vi "drive_to_wall.vi"(11 "NXT":T1) -> (3 "NXT 2":T1 caption="NXT")   [LabVIEW 2012]
uses:
  <vilib>/NXT/Subs/LVHSConnector.ctl
  <vilib>/NXT/Subs/MotorOutput.ctl
  <vilib>/NXT/Block Support/NXT_InputPort.ctl
  <vilib>/NXT/Dual Mode Library/Motors/MotorBrake.vi
  <vilib>/NXT/Dual Mode Library/prims/addArrayElements_int.vi
  <vilib>/NXT/Dual Mode Library/Motors/MotorReverse.vi
  <vilib>/NXT/Dual Mode Library/Waits/Wait_Num(msec).vi
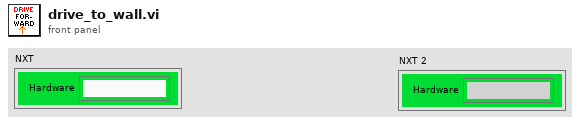
[diagram p1: front panel]
types:
  T1 = typedef "LVHSConnector.ctl" = cluster{"Hardware":string, "Flattened String":string}
  T2 = typedef "MotorOutput.ctl" = u8
  T3 = typedef "NXT_InputPort.ctl" = u8
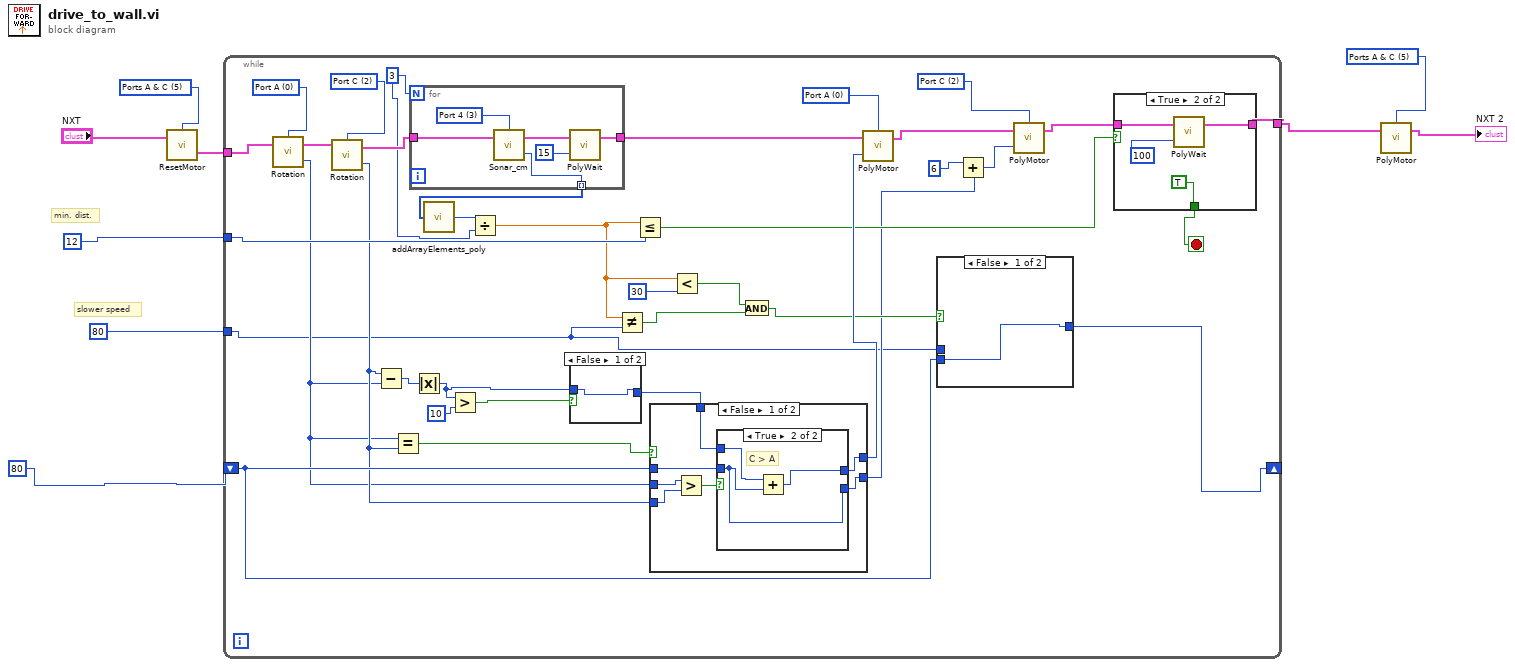
[diagram p0: block diagram]
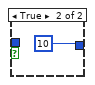
[diagram p2: hidden frame]
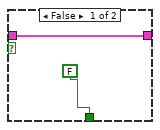
[diagram p4: hidden frame]
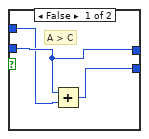
[diagram p5: hidden frame]
diagram:
  w9 = T2 5 items=["Port A"=0, "Port B"=1, "Port C"=2, "Ports A & B"=4, "Ports A & C"=5, "Ports B & C"=6, "All Ports"=3] ("Output Port (All Ports)")
  w7 = T2 5 items=["Port A"=0, "Port B"=1, "Port C"=2, "Ports A & B"=4, "Ports A & C"=5, "Ports B & C"=6, "All Ports"=3] ("Output Port (All Ports)")
  # "min. dist."
  # "slower speed"
  n1 = call <vilib>:"ResetMotor.vi"("NXT"="NXT", "Port (All Ports)"=w7) -> ("NXT"=w8:T1)  [unwired: 2 in]
  n2 = while {
    tunnel: w8 -> [w46]
    tunnel: [w34] -> w6
    tunnel: 12 -> [w36]
    shift-right: [w26] -> _
    shift-left: 80 -> [w25]
    tunnel: 80 -> [w10]
    stop <- w31 stop-if-true
    w11 = 3
    w39 = T2 2 items=["Port A"=0, "Port B"=1, "Port C"=2, "Ports A & B"=4, "Ports A & C"=5, "Ports B & C"=6, "All Ports"=3] ("Output Port (All Ports)")
    w40 = T2 0 items=["Port A"=0, "Port B"=1, "Port C"=2, "Ports A & B"=4, "Ports A & C"=5, "Ports B & C"=6, "All Ports"=3] ("Output Port (All Ports)")
    w41 = T2 2 items=["Port A"=0, "Port B"=1, "Port C"=2, "Ports A & B"=4, "Ports A & C"=5, "Ports B & C"=6, "All Ports"=3] ("Output Port (All Ports)")
    w42 = T2 0 items=["Port A"=0, "Port B"=1, "Port C"=2, "Ports A & B"=4, "Ports A & C"=5, "Ports B & C"=6, "All Ports"=3] ("Output Port (All Ports)")
    n3 = call <vilib>:"Rotation.vi"("NXT"=w46, "Port (Port A)"=w40) -> ("Angle of Rotation"=w23:i32, "NXT"=w45:T1)  [unwired: 1 in]
    n4 = call <vilib>:"Rotation.vi"("NXT"=w45, "Port (Port A)"=w39) -> ("Angle of Rotation"=w24:i32, "NXT"=w44:T1)  [unwired: 1 in]
    n5 = Subtract(x=w24, y=w23) -> (x-y=w22:i32)
    n6 = Equal?(x=w23, y=w24) -> (x = y?=w38:bool)
    n7 = for {
      N: w11 -> [_]
      tunnel: w44 -> [w51]
      tunnel: [w49] -> w37
      tunnel: [w50] -> w14 mode=indexing
      w52 = T3 3 items=["Port 1", "Port 2", "Port 3", "Port 4"] ("Port (Port 4)")
      n8 = call <vilib>:"Sonar_cm.vi"("NXT"=w51, "Port (Port 4)"=w52) -> ("Distance (cm)"=w50:i16, "NXT"=w48:T1)  [unwired: 1 in]
      n9 = call-poly <vilib>:"PolyWait.vi"("Time (100 msec)"=15, "NXT"=w48) -> ("NXT"=w49:T1)  [unwired: 2 in]
    }
    n10 = Absolute Value(x=w22) -> (abs(x)=w19:i32)
    n11 = call-poly <vilib>:"addArrayElements_poly.vi"("Numeric Array"=w14) -> ("Sum"=w13:i32)
    n12 = Greater?(x=w19, y=10) -> (0:w20:bool)
    n13 = Divide(x=w13, y=w11) -> (x/y=w12:dbl)
    n14 = case shown="False" w20 {
      tunnel: [w53 10] -> w18
      tunnel: w19 -> [w53 _]
      frame False {
      }
      frame True {
      }
    }
    n15 = Not Equal?(x=w12, y=w10) -> (x != y?=w28:bool)
    n16 = Less Or Equal?(x=w12, y=w36) -> (x <= y?=w32:bool)
    n17 = case shown="False" w38 {
      tunnel: [w67 w76] -> w35
      tunnel: w25 -> [w68 w76]
      tunnel: [w66 w76] -> w16
      tunnel: w24 -> [w65 _]
      tunnel: w23 -> [w64 _]
      tunnel: w18 -> [w63 _]
      frame False {
        n18 = Greater?(x=w64, y=w65) -> (0:w69:bool)
        n19 = case shown="True" w69 {
          tunnel: w68 -> [w71 w75]
          tunnel: [w71 w73] -> w67
          tunnel: [w72 w75] -> w66
          tunnel: w63 -> [w70 w74]
          frame False {
            # "A > C"
            n20 = Add(x=w71, y=w70) -> (x+y=w72:i32)
          }
          frame True {
            # "C > A"
            n21 = Add(x=w74, y=w75) -> (x+y=w73:i32)
          }
        }
      }
      frame True {
      }
    }
    n22 = Less?(x=w12, y=30) -> (x < y?=w29:bool)
    n23 = And(x=w29, y=w28) -> (x .and. y?=w27:bool)
    n24 = call-poly <vilib>:"PolyMotor.vi"("Power (75)"=w35, "NXT"=w37, "Output Port (All Ports)"=w42) -> ("NXT"=w43:T1)  [unwired: 1 in]
    n25 = case shown="False" w27 {
      tunnel: [w55 w56] -> w26
      tunnel: w25 -> [w55 _]
      tunnel: w10 -> [_ w56]
      frame False {
      }
      frame True {
      }
    }
    n26 = Add(x=6, y=w16) -> (x+y=w15:i32)
    n27 = call-poly <vilib>:"PolyMotor.vi"("Power (75)"=w15, "NXT"=w43, "Output Port (All Ports)"=w41) -> ("NXT"=w33:T1)  [unwired: 1 in]
    n28 = case shown="True" w32 {
      tunnel: [w57 w62] -> w34
      tunnel: w33 -> [w57 w60]
      tunnel: [FALSE TRUE] -> w31
      frame False {
      }
      frame True {
        n29 = call-poly <vilib>:"PolyWait.vi"("Time (100 msec)"=100, "NXT"=w60) -> ("NXT"=w62:T1)  [unwired: 2 in]
      }
    }
  }
  n30 = call-poly <vilib>:"PolyMotor.vi"("NXT"=w6, "Port (All Ports)"=w9) -> ("NXT"=→"NXT 2":T1)  [unwired: 2 in]
